vi "Add exp.vi"(8 "error in (no error)":errorcluster, 10 "New exp":refnum<class "Experiment.lvclass">, 11 "Experiments_group in":refnum<class "Experiments_group.lvclass">) -> (0 "error out":errorcluster, 3 "Experiments_group out":refnum<class "Experiments_group.lvclass">)   [LabVIEW 2015, in "Experiments_group.lvclass"]
uses:
  Experiments_group.lvclass
  Experiment.lvclass
  Experiments_group.lvclass/Experiments_group.ctl
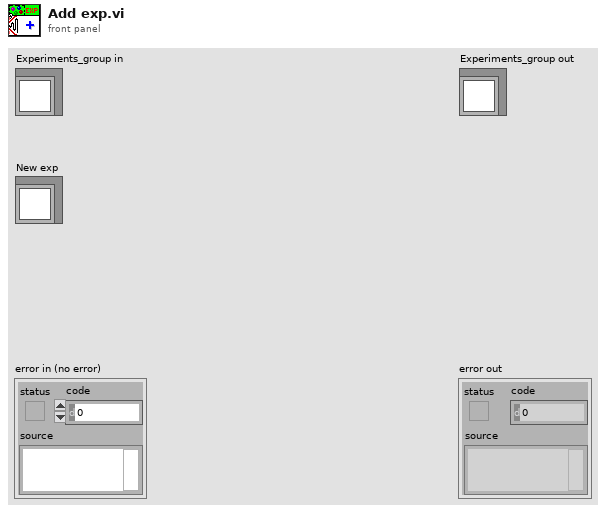
[diagram p1: front panel]
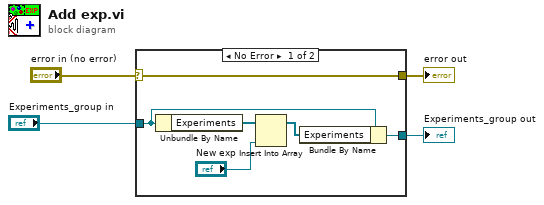
[diagram p0: block diagram]
diagram:
  n1 = case shown="No Error" "error in (no error)" {
    selector: "error in (no error)" -> [w10 w12]
    tunnel: [w10 w12] -> w3
    tunnel: [w8 w11] -> w1
    tunnel: "Experiments_group in" -> [w9 w11]
    frame No Error {
      n2 = Unbundle By Name(w9) -> ("Experiments"=w7:refnum<class "Experiment.lvclass">[])
      n3 = Insert Into Array(array=w7, new element="New exp") -> (w5:refnum<class "Experiment.lvclass">[])  [unwired: 1 in]
      n4 = Bundle By Name(cluster=w9, "Experiments"=w5) -> (w8:refnum<class "Experiments_group.lvclass">)
    }
    frame Error {
    }
  }
  "error out" <- w3
  "Experiments_group out" <- w1
